vi "full parse.vi"(8 "query delimiter":string="&", 9 "default port":u16, 10 "path delimiter":string="/", 11 "URL string":string) -> (3 "URL":T1)   [LabVIEW 2013, in "uniform resource locator.lvlib"]
uses:
  uniform resource locator.lvlib
  url structure.ctl
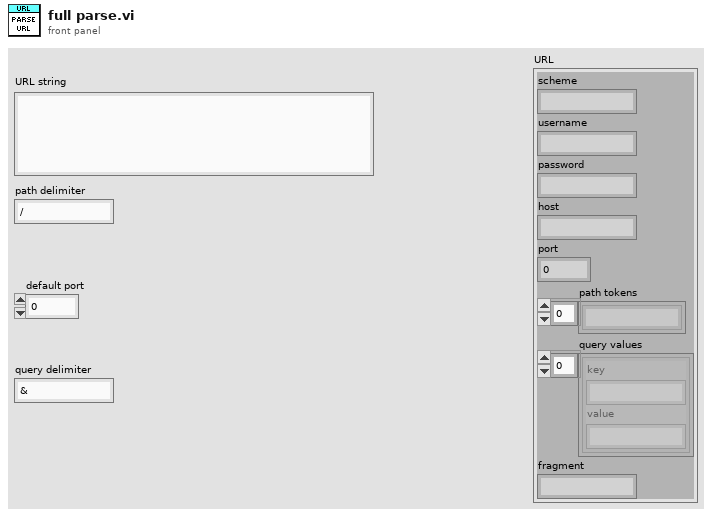
[diagram p1: front panel]
types:
  T1 = typedef "uniform resource locator.lvlib/url structure.ctl" = cluster{"scheme":string, "username":string, "password":string, "host":string, "port":u16, "path tokens":string[], "query values":cluster{"key":string, "value":string}[], "fragment":string}
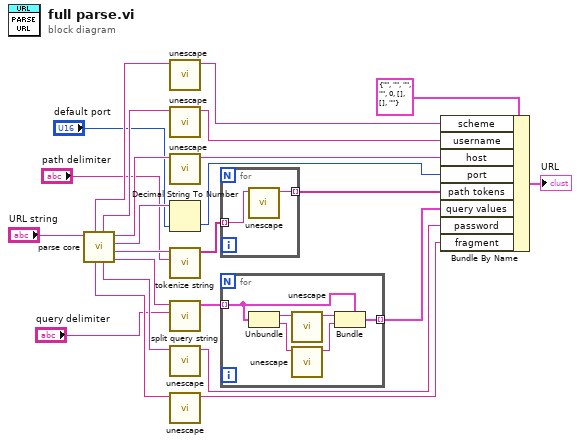
[diagram p0: block diagram]
diagram:
  n1 = call "parse core.vi"("URL"="URL string") -> ("query"=w4:string, "path"=w8:string, "port"=w11:string, "host"=w13:string, "password"=w19:string, "username"=w15:string, "fragment"=w21:string, "scheme"=w16:string)  [unwired: 3 in]
  n2 = call "unescape.vi"("escaped string"=w16) -> ("unescaped"=w17:string)  [unwired: 10 in]
  n3 = call "unescape.vi"("escaped string"=w15) -> ("unescaped"=w14:string)  [unwired: 10 in]
  n4 = call "unescape.vi"("escaped string"=w13) -> ("unescaped"=w12:string)  [unwired: 10 in]
  n5 = Decimal String To Number(string=w11, default (0L)="default port") -> (number=w9:u16)  [unwired: 1 in, 1 out]
  n6 = call "tokenize string.vi"("delimiter"="path delimiter", "raw path"=w8) -> ("segments"=w6:string[])  [unwired: 9 in]
  n7 = call "split query string.vi"("delimiter"="query delimiter", "query"=w4) -> ("query values"=w2:cluster{"key":string, "value":string}[])  [unwired: 9 in]
  n8 = call "unescape.vi"("escaped string"=w19) -> ("unescaped"=w18:string)  [unwired: 10 in]
  n9 = call "unescape.vi"("escaped string"=w21) -> ("unescaped"=w20:string)  [unwired: 10 in]
  n10 = for {
    tunnel: w6 -> [w26] mode=indexing
    tunnel: [w25] -> w5 mode=indexing
    n11 = call "unescape.vi"("escaped string"=w26) -> ("unescaped"=w25:string)  [unwired: 10 in]
  }
  n12 = for {
    tunnel: w2 -> [w32] mode=indexing
    tunnel: [w31] -> w1 mode=indexing
    n13 = Unbundle(w32) -> ("key"=w30:string, "value"=w29:string)
    n14 = call "unescape.vi"("escaped string"=w30) -> ("unescaped"=w27:string)  [unwired: 10 in]
    n15 = call "unescape.vi"("escaped string"=w29) -> ("unescaped"=w28:string)  [unwired: 10 in]
    n16 = Bundle(cluster=w32, "key"=w27, "value"=w28) -> (w31:cluster{"key":string, "value":string})
  }
  n17 = Bundle By Name(cluster=T1 {"scheme"="", "username"="", "password"="", "host"="", "port"=0, "path tokens"=[], "query values"=[], "fragment"=""} ("URL"), "scheme"=w17, "username"=w14, "host"=w12, "port"=w9, "path tokens"=w5, "query values"=w1, "password"=w18, "fragment"=w20) -> (→"URL":T1)
